vi "mlink_ai_scan_init.vi"(5 "range":dbl[](array[numeric]), 6 "channels":u8[](array[numeric]), 7 "mode":T1[](array[typedef]), 8 "error in (no error)":errorcluster, 9 "rate":sgl, 10 "duration":sgl, 11 "connection ID":i32=-1) -> (0 "error out":errorcluster, 1 "actual rate":sgl, 3 "connection ID out":i32)   [LabVIEW 2009, in "MicroDAQ.lvlib" / "mlink.lvlib"]
doc: "This function initiates analog input scanning session. The function must be called before \nacquisition started. The channels argument is an array containing channels numbers according to MicroDAQ hardware configuration. The ch_count argument determines number of used channels. The range argument specifies channel measurement input range. An array n-by-2 where n is number of used channels shall be provided. In order to obtain supported ranges check your ADC configuration. The mode argument specifies measurement mode - differential or single-ended. An mode array of mode settings for used channels shall be provided.\nThe rate argument determines scans per second rate for selected analog input channels. \nMinimum value is 1 scan per second, maximum depends on MicroDAQ analog input type.\nThe duration argument specifies a duration of acquisition in seconds. When set to -1, the \nsession will run continuously, acquiring data until stopped with mlink_ai_scan_stop() function call."
uses:
  <instrlib>/MicroDAQ/Mlink library wraper/mlink.lvlib
  <instrlib>/MicroDAQ/Tools/Analog input type enum.ctl
  <instrlib>/MicroDAQ/MLink32.dll
  <instrlib>/MicroDAQ/MicroDAQ.lvlib
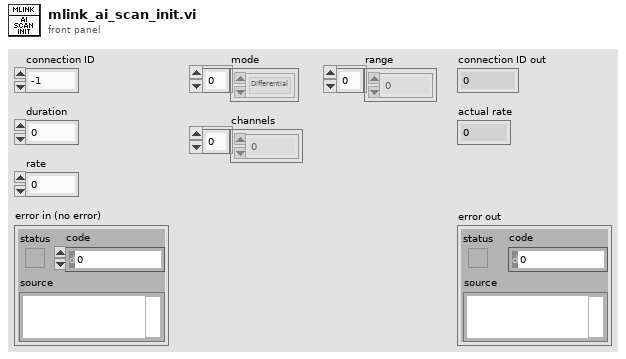
[diagram p1: front panel]
types:
  T1 = typedef "MicroDAQ.lvlib/Analog input type enum.ctl" = enum8{"Single-ended", "Differential"}
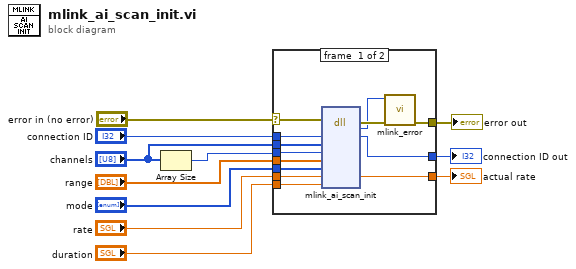
[diagram p0: block diagram]
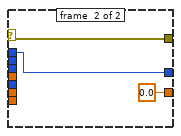
[diagram p2: hidden frame]
diagram:
  n1 = Array Size(array="channels") -> (size(s)=w5:i32)
  n2 = case shown="No Error" "error in (no error)" {
    selector: "error in (no error)" -> [w22 w26]
    tunnel: "connection ID" -> [w24 w27]
    tunnel: [w23 w27] -> w10
    tunnel: "rate" -> [w21 _]
    tunnel: "duration" -> [w20 _]
    tunnel: [w19 sgl 0.0 ("rate")] -> w6
    tunnel: w5 -> [w18 _]
    tunnel: "mode" -> [w17 _]
    tunnel: "range" -> [w16 _]
    tunnel: "channels" -> [w15 _]
    tunnel: [w12 w26] -> w1
    frame #0 {
      n3 = dll-call lib="C:/Program Files (x86)/National Instruments/LabVIEW 2009/instr.lib/MicroDAQ/MLink32.dll" fn="mlink_ai_scan_init"(error in=w22, "connection ID"=w24, "channels"=w15, "count"=w18, "range"=w16, "mode"=w17, "rate"=w21, "duration"=w20) -> (error out=w14:errorcluster, "return type"=w13:i32, "connection ID"=w23:i32, "rate"=w19:sgl)  [unwired: 7 in, 1 out]
      n4 = call <instrlib>:"mlink_error.vi"("error in (no error)"=w14, "error code"=w13) -> ("error out"=w12:errorcluster)  [unwired: 9 in]
    }
    frame #1 {
    }
  }
  "connection ID out" <- w10
  "actual rate" <- w6
  "error out" <- w1
